vi "PH_BackreflectionMeas.Save Data 2 Harddisk.vi"(0 "i ref in":refnum<vi>, 5 "error in":errorcluster) -> (14 "i ref out":refnum<vi>, 19 "error out":errorcluster)   [LabVIEW 2014, in "PH_BackreflectionMeas.lvlib"]
uses:
  PH_BackreflectionMeas.lvlib
  PH_Common/PH_Common.lvlib
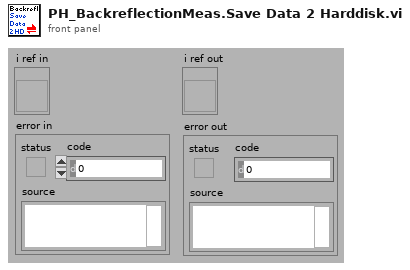
[diagram p1: front panel]
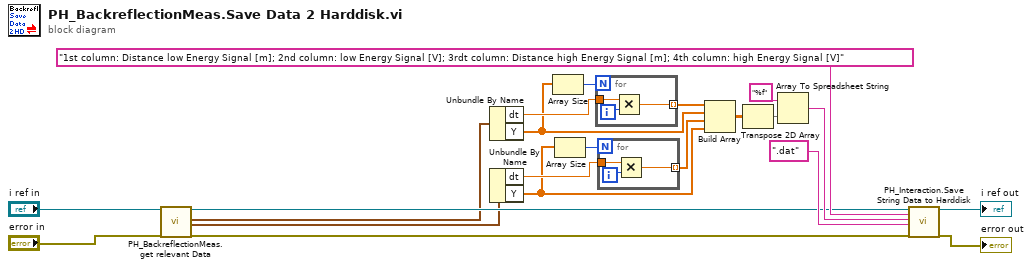
[diagram p0: block diagram]
diagram:
  n1 = call "PH_BackreflectionMeas.get relevant Data.vi"("i ref in"="i ref in", "error in"="error in") -> ("i ref out"=w5:refnum<vi>, "low Energy Waveform"=w2:waveform(dbl), "high Energy Waveform"=w1:waveform(dbl), "error out"=w3:errorcluster)  [unwired: 14 in]
  n2 = Unbundle By Name(w2) -> ("dt"=w17:dbl, "Y"=w12:dbl[])
  n3 = Unbundle By Name(w1) -> ("dt"=w15:dbl, "Y"=w14:dbl[])
  n4 = Array Size(array=w12) -> (size(s)=w18:i32)
  n5 = Array Size(array=w14) -> (size(s)=w16:i32)
  n6 = for {
    N: w18 -> [_]
    tunnel: w17 -> [w25]
    tunnel: [w23] -> w22 mode=indexing
    i -> [w24]
    n7 = Multiply(x=w25, y=w24) -> (x*y=w23:dbl)
  }
  n8 = for {
    N: w16 -> [_]
    tunnel: w15 -> [w28]
    tunnel: [w26] -> w13 mode=indexing
    i -> [w27]
    n9 = Multiply(x=w28, y=w27) -> (x*y=w26:dbl)
  }
  n10 = Build Array(w22, w12, w13, w14) -> (w21:dbl[][])
  n11 = Transpose 2D Array(2D array=w21) -> (transposed array=w20:dbl[][])
  n12 = Array To Spreadsheet String(array=w20, 3:"%f" ("format string")) -> (spreadsheet string=w10:string)  [unwired: 1 in]
  n13 = call "PH_Interaction.Save String Data to Harddisk.vi"("i ref in"=w5, "Explanation (for Example: Column 1: xxx, ...)"="1st column: Distance low Energy Signal [m]; 2nd column: low Energy Signal [V]; 3rdt column: Distance high Energy Signal [m]; 4th column: high Energy Signal [V]" ("string"), "Data (for example: Columns)"=w10, "file name extension"=".dat" ("file name extinction"), "error in (no error)"=w3) -> ("i ref out"=→"i ref out":refnum<vi>, "error out"=→"error out":errorcluster)  [unwired: 12 in, 1 out]
